vi "Set Event Capture Properties.vi"(8 "error in (no error)":errorcluster, 10 "capture":T1={"Name"="", "Bitfile name"="", "Reference angle"=0.0, "Default start"=-90.0, "Default end"=-90.0, "Ref Select"=enum."From window"}, 11 "Item Ref in":T3 format="%.0x") -> (0 "error out":errorcluster, 2 "failed":bool, 3 "Item Ref out":T3 format="%.0x")   [LabVIEW 2017, in "Engine Simulation Toolkit System Explorer.lvlib"]
uses:
  Engine Simulation Toolkit System Explorer.lvlib
  <vilib>/NI Veristand/Custom Device API/Custom Device Item Ref.ctl
  Event Timing Capture.ctl
  Event Reference Angle Selection.ctl
  Shared/Properties.vi
  <vilib>/NI Veristand/Custom Device Tools/Custom Device Utility Library/NI VeriStand - Search for Item by Property.vi
  <vilib>/NI Veristand/Custom Device API/Set Item Property (Double).vi
  <vilib>/NI Veristand/Custom Device API/Set Item Property (U16).vi
  <vilib>/NI Veristand/Custom Device API/Custom Device API.lvlib
  Shared/Engine Simulation Toolkit Shared.lvlib
  <vilib>/NI Veristand/Custom Device Tools/Custom Device Utility Library/Custom Device Utility Library.lvlib
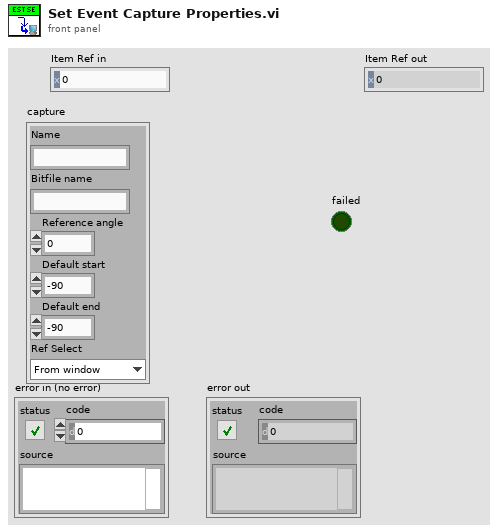
[diagram p1: front panel]
types:
  T1 = typedef "Engine Simulation Toolkit System Explorer.lvlib/Event Timing Capture.ctl" = cluster{"Name":string, "Bitfile name":string, "Reference angle":dbl, "Default start":dbl, "Default end":dbl, "Ref Select":T2}
  T2 = typedef "Engine Simulation Toolkit System Explorer.lvlib/Event Reference Angle Selection.ctl" = enum16{"From window", "Custom"}
  T3 = typedef "Custom Device API.lvlib/Custom Device Item Ref.ctl" = u64
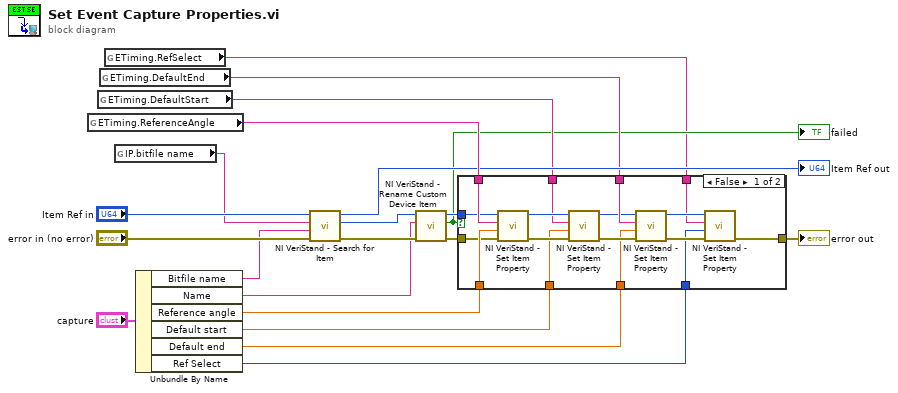
[diagram p0: block diagram]
diagram:
  n1 = global read "Properties.vi" "ETiming.ReferenceAngle"() -> (w19:string)
  n2 = global read "Properties.vi" "ETiming.DefaultStart"() -> (w12:string)
  n3 = global read "Properties.vi" "ETiming.DefaultEnd"() -> (w5:string)
  n4 = global read "Properties.vi" "ETiming.RefSelect"() -> (w1:string)
  n5 = global read "Properties.vi" "IP.bitfile name"() -> (w10:string)
  n6 = Unbundle By Name("capture") -> ("Bitfile name"=w11:string, "Name"=w6:string, "Reference angle"=w14:dbl, "Default start"=w13:dbl, "Default end"=w4:dbl, "Ref Select"=w2:T2)
  n7 = call-poly <vilib>:"NI VeriStand - Search for Item.vi"("error in"="error in (no error)", "Property Value"=w11, "Property Name"=w10, "Section Ref in"="Item Ref in") -> ("error out"=w17:errorcluster, "Item Ref"=w8:T3, "Section Ref out"=→"Item Ref out":T3)  [unwired: 4 in, 1 out]
  n8 = call <vilib>:"NI VeriStand - Rename Custom Device Item.vi"("error in (no error)"=w17, "New Name"=w6, "Item Ref in"=w8) -> ("error out"=w9:errorcluster, "Request invalid?"=w3:bool, "Item Ref out"=w7:T3)  [unwired: 6 in]
  "failed" <- w3
  n9 = case shown="False" w3 {
    tunnel: [w24 w39] -> w20
    tunnel: w19 -> [w35 _]
    tunnel: w14 -> [w34 _]
    tunnel: w13 -> [w33 _]
    tunnel: w12 -> [w32 _]
    tunnel: w9 -> [w31 w39]
    tunnel: w7 -> [w30 _]
    tunnel: w5 -> [w29 _]
    tunnel: w4 -> [w27 _]
    tunnel: w2 -> [w23 _]
    tunnel: w1 -> [w22 _]
    frame False {
      n10 = call-poly <vilib>:"NI VeriStand - Set Item Property.vi"("error in (no error)"=w31, "Value"=w34, "Property Name"=w35, "Item Ref in"=w30) -> ("error out"=w38:errorcluster, "Item Ref out"=w36:T3)  [unwired: 5 in, 1 out]
      n11 = call-poly <vilib>:"NI VeriStand - Set Item Property.vi"("error in (no error)"=w38, "Value"=w33, "Property Name"=w32, "Item Ref in"=w36) -> ("error out"=w37:errorcluster, "Item Ref out"=w28:T3)  [unwired: 5 in, 1 out]
      n12 = call-poly <vilib>:"NI VeriStand - Set Item Property.vi"("error in (no error)"=w37, "Value"=w27, "Property Name"=w29, "Item Ref in"=w28) -> ("error out"=w25:errorcluster, "Item Ref out"=w26:T3)  [unwired: 5 in, 1 out]
      n13 = call-poly <vilib>:"NI VeriStand - Set Item Property.vi"("error in (no error)"=w25, "Value"=w23, "Property Name"=w22, "Item Ref in"=w26) -> ("error out"=w24:errorcluster)  [unwired: 5 in, 2 out]
    }
    frame True {
    }
  }
  "error out" <- w20
